vi "Read Fiducial Parameters.vi"(8 "error in":errorcluster, 10 "Fiducial Type":T1, 11 "Config Manager in":refnum<class "Config Manager Class.lvclass">) -> (0 "error out":errorcluster, 1 "Interactive Mode":bool, 2 "Fiducial Parameters":T2, 3 "Config Manager out":refnum<class "Config Manager Class.lvclass">)   [LabVIEW 2011, in "Config Manager Class.lvclass"]
uses:
  Config Manager Class.lvclass
  Type Definitions/Fiducial Finder Parameters.ctl
  Type Definitions/Fiducial Type.ctl
  Config Manager Class.lvclass/Config Manager Class.ctl
  <vilib>/Utility/config.llb/Read Key (Boolean).vi
  <vilib>/Utility/config.llb/Read Key (I32).vi
  <vilib>/Utility/config.llb/Read Key (Double).vi
  <vilib>/Utility/config.llb/NI_LVConfig.lvlib
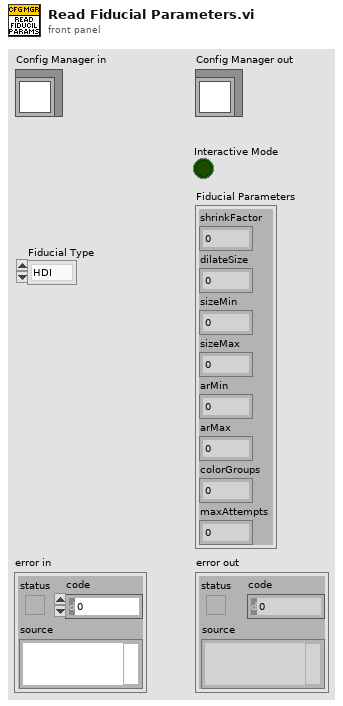
[diagram p1: front panel]
types:
  T1 = typedef "Fiducial Type.ctl" = enum16{"HDI", "BBM"}
  T2 = typedef "Fiducial Finder Parameters.ctl" = cluster{"shrinkFactor":sgl, "dilateSize":i32, "sizeMin":sgl, "sizeMax":sgl, "arMin":sgl, "arMax":sgl, "colorGroups":i32, "maxAttempts":i32}
  T3 = typedef "NI_LVConfig.lvlib/Config Data RefNum.ctl" = refnum<k1>
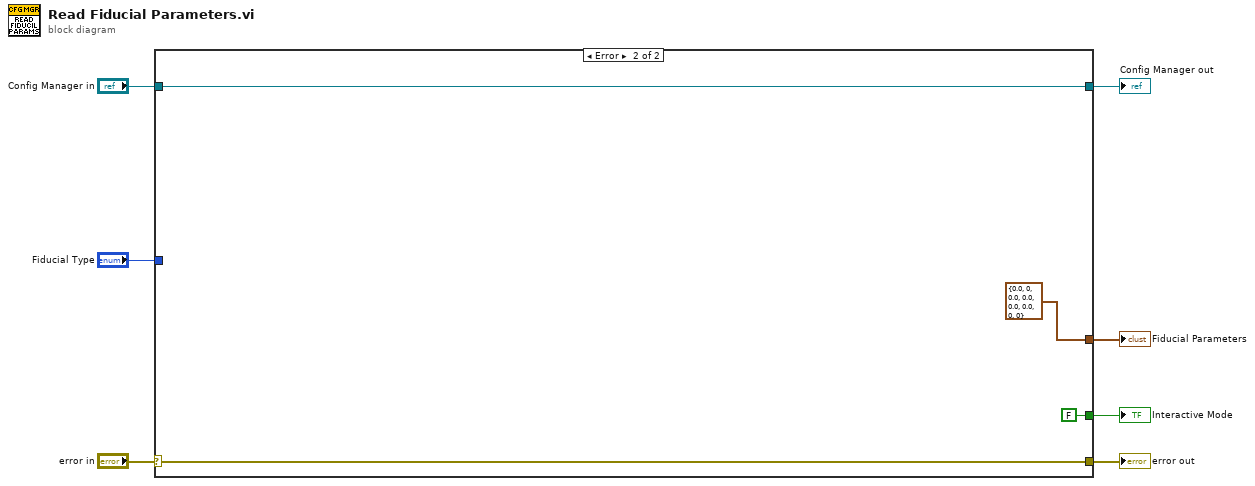
[diagram p0: block diagram]
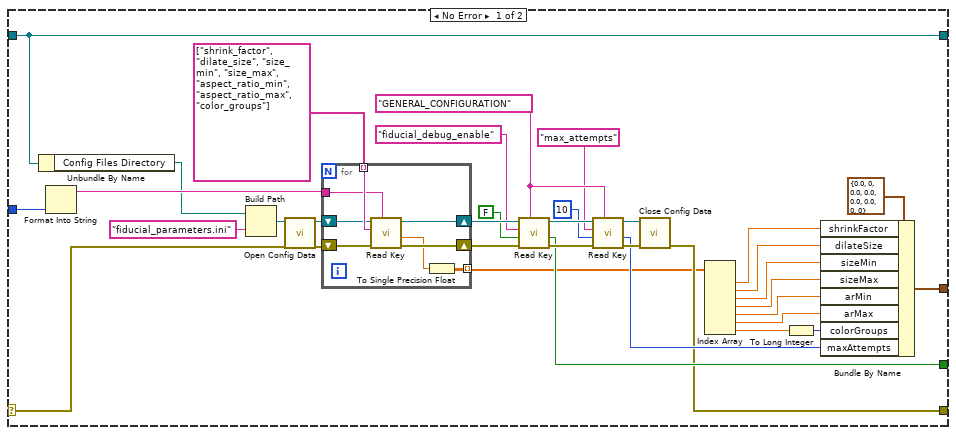
[diagram p2: hidden frame]
diagram:
  n1 = case shown="Error" "error in" {
    selector: "error in" -> [w12 w54]
    tunnel: [w11 w54] -> w6
    tunnel: [w16 w53] -> w4
    tunnel: "Config Manager in" -> [w16 w53]
    tunnel: [w18 T2 {"shrinkFactor"=0.0, "dilateSize"=0, "sizeMin"=0.0, "sizeMax"=0.0, "arMin"=0.0, "arMax"=0.0, "colorGroups"=0, "maxAttempts"=0} ("Fiducial Parameters")] -> w3
    tunnel: [w17 FALSE ("value")] -> w2
    tunnel: "Fiducial Type" -> [w15 _]
    frame No Error {
      w22 = "GENERAL_CONFIGURATION" ("section")
      n2 = Unbundle By Name(w16) -> ("Config Files Directory"=w13:path)
      n3 = Format Into String(w15) -> (resulting string=w14:string)  [unwired: 3 in, 1 out]
      n4 = Build Path(base path=w13, name or relative path="fiducial_parameters.ini") -> (appended path=w41:path)
      n5 = call <vilib>:"Open Config Data.vi"("error in (no error)"=w12, "configuration file path"=w41) -> ("error out"=w39:errorcluster, "refnum"=w38:T3)  [unwired: 7 in, 1 out]
      n6 = for {
        tunnel: string[] ["shrink_factor", "dilate_size", "size_min", "size_max", "aspect_ratio_min", "aspect_ratio_max", "color_groups"] -> [w50] mode=indexing
        tunnel: w14 -> [w49]
        shift-right: [w47] -> w36
        shift-left: w39 -> [w48]
        shift-right: [w45] -> w37
        shift-left: w38 -> [w46]
        tunnel: [w43] -> w10 mode=indexing
        n7 = call-poly <vilib>:"Read Key.vi"("section"=w49, "error in (no error)"=w48, "key"=w50, "refnum"=w46) -> ("error out"=w47:errorcluster, "value"=w44:dbl, "refnum out"=w45:T3)  [unwired: 4 in, 1 out]
        n8 = To Single Precision Float(number=w44) -> (single precision float=w43:sgl)
      }
      n9 = call-poly <vilib>:"Read Key.vi"("section"=w22, "error in (no error)"=w36, "default value"=FALSE, "key"="fiducial_debug_enable", "refnum"=w37) -> ("error out"=w25:errorcluster, "value"=w17:bool, "refnum out"=w26:T3)  [unwired: 3 in, 1 out]
      n10 = call-poly <vilib>:"Read Key.vi"("section"=w22, "error in (no error)"=w25, "default value"=10, "key"="max_attempts", "refnum"=w26) -> ("error out"=w23:errorcluster, "value"=w20:i32, "refnum out"=w24:T3)  [unwired: 3 in, 1 out]
      n11 = call <vilib>:"Close Config Data.vi"("error in (no error)"=w23, "refnum"=w24) -> ("error out"=w11:errorcluster)  [unwired: 8 in, 1 out]
      n12 = Index Array(array=w10) -> (element #1=w33:sgl, element #2=w32:sgl, element #3=w31:sgl, element #4=w30:sgl, element #5=w29:sgl, element #6=w28:sgl, element #7=w9:sgl)  [unwired: 7 in]
      n13 = To Long Integer(number=w9) -> (32bit integer=w8:i32)
      n14 = Bundle By Name(cluster=T2 {"shrinkFactor"=0.0, "dilateSize"=0, "sizeMin"=0.0, "sizeMax"=0.0, "arMin"=0.0, "arMax"=0.0, "colorGroups"=0, "maxAttempts"=0} ("Fiducial Parameters"), "shrinkFactor"=w33, "dilateSize"=w32, "sizeMin"=w31, "sizeMax"=w30, "arMin"=w29, "arMax"=w28, "colorGroups"=w8, "maxAttempts"=w20) -> (w18:T2)
    }
    frame Error {
    }
  }
  "error out" <- w6
  "Config Manager out" <- w4
  "Fiducial Parameters" <- w3
  "Interactive Mode" <- w2
